vi "PrepareIESource.vi"(10 "Manual Test":bool) -> (0 "error out":errorcluster)   [LabVIEW 2020]
uses:
  <vilib>/Wiresmith Technology/G CLI/CLI Class/CLI.lvclass
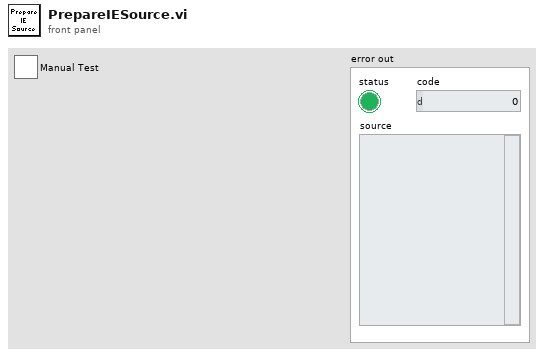
[diagram p1: front panel]
types:
  T1 = enum32{"Invalid", "Standard", "Closed", "Hidden", "Minimized", "Maximized"}
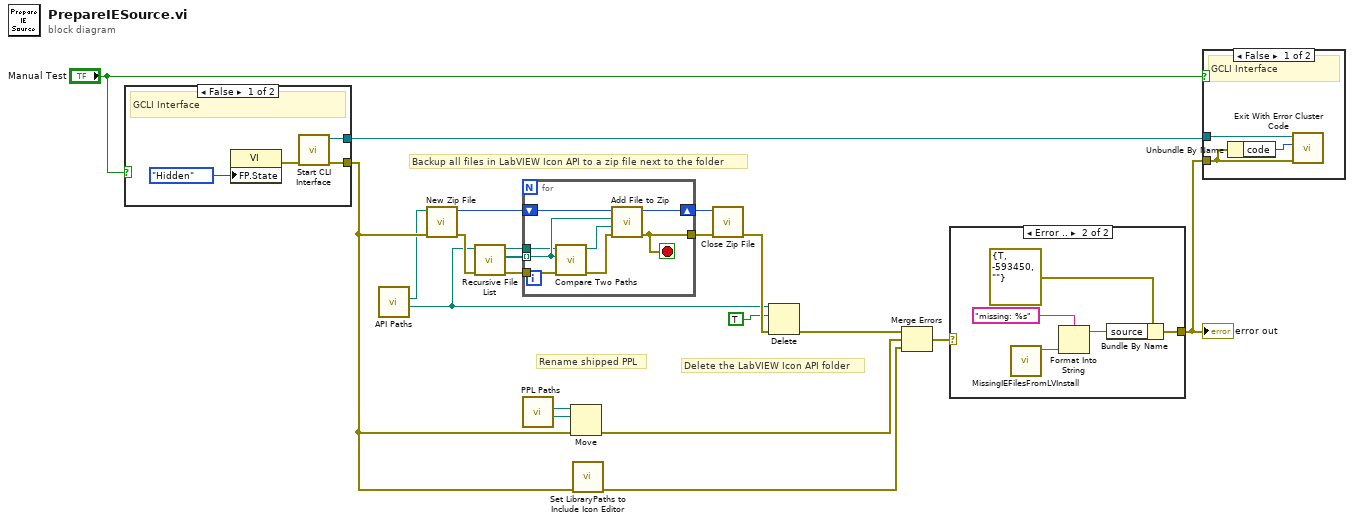
[diagram p0: block diagram]
diagram:
  # "Rename shipped PPL"
  # "Delete the LabVIEW Icon API folder"
  # "Backup all files in LabVIEW Icon API to a zip file next to the folder"
  n1 = case shown="False" "Manual Test" {
    tunnel: [w24 _] -> w17
    tunnel: [w22 _] -> w10
    frame False {
      # "GCLI Interface"
      n2 = property class="VI"("FP.State"=T1."Hidden" ("Front Panel Window:State")) -> (error out=w25:errorcluster)  [unwired: 2 in, 1 out]
      n3 = call <vilib>:"Start CLI Interface.vi"("error in (no error)"=w25) -> ("error out"=w24:errorcluster, "CLI out"=w22:refnum<class "CLI.lvclass">)  [unwired: 7 in, 2 out]
    }
    frame True {
      # "Running Manual"
    }
  }
  n4 = call "API Paths.vi"() -> ("API Folder"=w3:path, "API Zip File"=w4:path)  [unwired: 10 in]
  n5 = call <vilib>:"New Zip File.vi"("error in (no error)"=w17, "target"=w4) -> ("error out"=w18:errorcluster, "zip file out"=w7:i64)  [unwired: 3 in, 1 out]
  n6 = call <vilib>:"Recursive File List.vi"("error in (no error)"=w18, "Folder Path"=w3) -> ("error out"=w19:errorcluster, "All Files in Dir"=w9:path[], "dup Folder Path"=w5:path)  [unwired: 5 in, 2 out]
  n7 = for {
    tunnel: w9 -> [w28] mode=indexing
    tunnel: w19 -> [w32]
    tunnel: [w33] -> w20
    shift-right: [w29] -> w8
    shift-left: w7 -> [w30]
    tunnel: w5 -> [w27]
    stop <- w33 stop-if-true
    n8 = call <vilib>:"Compare Two Paths.vi"("error in (no error)"=w32, "Path 2"=w28, "Path 1"=w27) -> ("error out"=w31:errorcluster, "Relative Path from 1 to 2"=w26:path)  [unwired: 5 in, 2 out]
    n9 = call <vilib>:"Add File to Zip.vi"("error in (no error)"=w31, "destination path in zip"=w26, "source file path"=w28, "zip file in"=w30) -> ("error out"=w33:errorcluster, "zip file out"=w29:i64)  [unwired: 6 out]
  }
  n10 = call "PPL Paths.vi"() -> ("Renamed PPL Path"=w1:path, "PPL Path"=w2:path)  [unwired: 10 in]
  n11 = Move(source path=w2, error in=w17, 10:w1) -> (error out=w15:errorcluster)  [unwired: 2 in, 2 out]
  n12 = call "Set LibraryPaths to Include Icon Editor.vi"("error in"=w17) -> ("error out"=w14:errorcluster)  [unwired: 9 in, 1 out]
  n13 = call <vilib>:"Close Zip File.vi"("error in (no error)"=w20, "zip file in"=w8) -> ("error out"=w21:errorcluster)  [unwired: 5 in]
  n14 = Delete(path (use dialog)=w3, entire hierarchy (F)=TRUE, error in=w21) -> (error out=w16:errorcluster)  [unwired: 2 in, 2 out]
  n15 = Merge Errors(w16, w15, w14) -> (w13:errorcluster)
  n16 = case shown="Error .." w13 {
    selector: w13 -> [w34 _]
    tunnel: [w34 w38] -> w12
    frame No Error {
    }
    frame Error {
      n17 = call "MissingIEFilesFromLVInstall.vi"() -> ("Missing IE Paths"=w35:string)  [unwired: 10 in, 1 out]
      n18 = Format Into String(format string="missing: %s", w35) -> (resulting string=w37:string)  [unwired: 2 in, 1 out]
      n19 = Bundle By Name(cluster=errorcluster {"status"=TRUE, "code"=-593450, "source"=""} ("error out"), "source"=w37) -> (w38:errorcluster)
    }
  }
  "error out" <- w12
  n20 = case shown="False" "Manual Test" {
    tunnel: w10 -> [w41 _]
    tunnel: w12 -> [w42 _]
    frame False {
      # "GCLI Interface"
      n21 = Unbundle By Name(w42) -> ("code"=w40:i32)
      n22 = call <vilib>:"Exit With Error Cluster Code.vi"("error in (no error)"=w42, "No Error Code (0)"=w40, "CLI in"=w41) -> ()  [unwired: 8 in, 1 out]
    }
    frame True {
      # "Running Manual"
    }
  }
